vi "PV reconnect.vi"(10 "Input cluster":T1) -> (0 "Vlim":bool, 1 "flim":bool, 2 "failure_flag 3":bool)   [LabVIEW 2016]
uses:
  Communication/Global communication.vi
  Communication/Global communication output.vi
panel:
  out "ready? 2":bool
  out "Boolean":bool
  in  "Max_2":bool
  in  "Max_2":bool
  in  "Max_1":bool
  in  "Max?":bool
  in  "Vlim?":bool
  in  "flim?":bool
  in  "ready?":bool
  in  "i>=20?":bool
  in  "=1?":bool
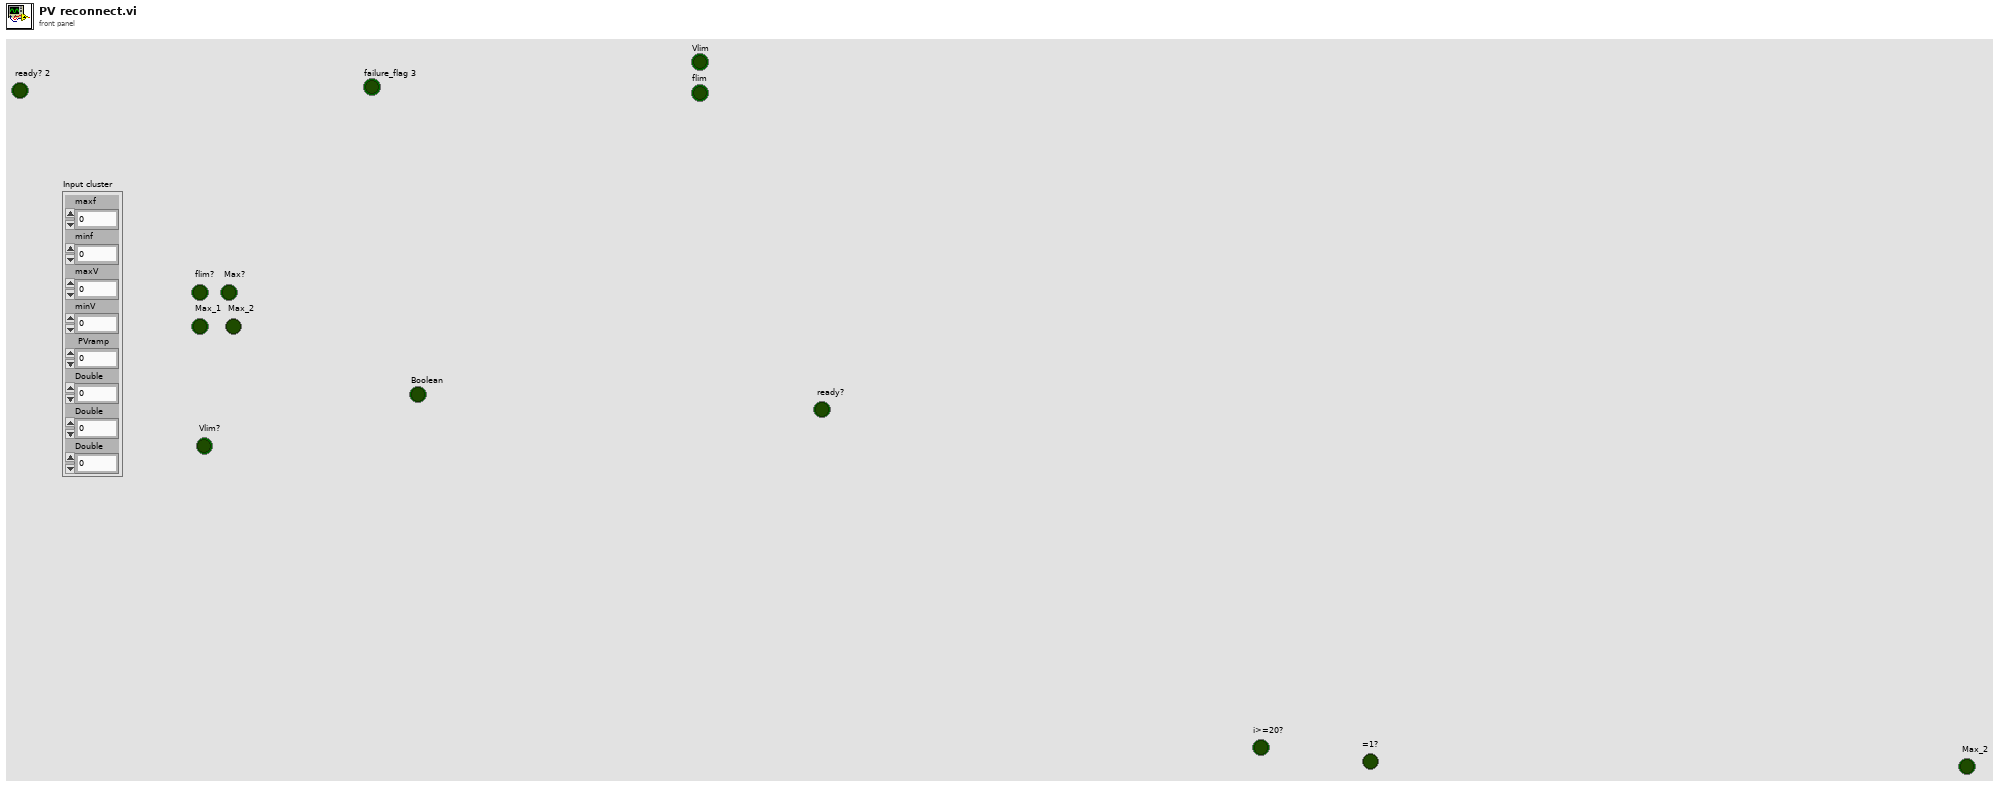
[diagram p1: front panel]
types:
  T1 = cluster{"maxf":dbl, "minf":dbl, "maxV":dbl, "minV":dbl, " PVramp":dbl, "Double":dbl, "Double":dbl, "Double":dbl}
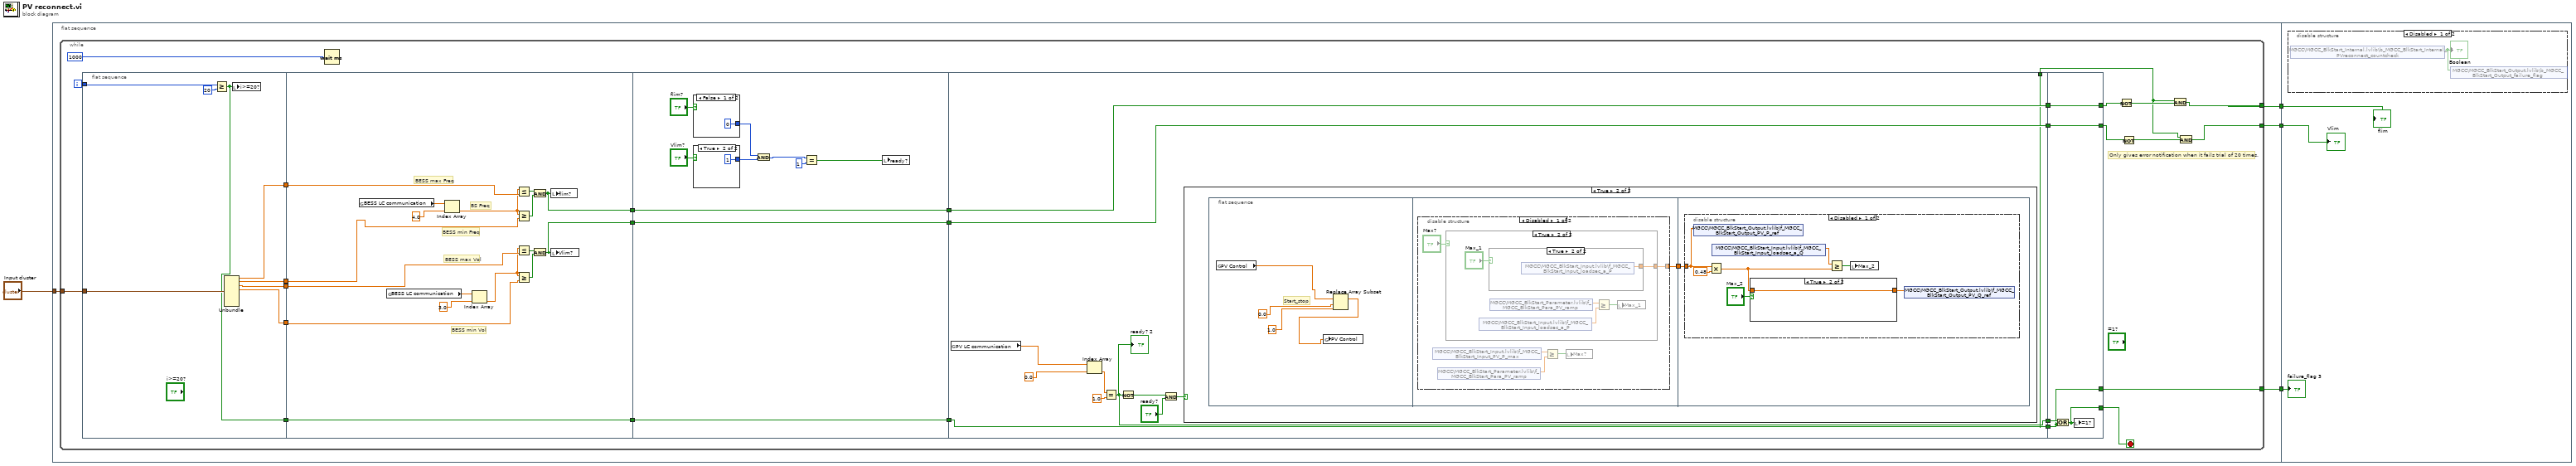
[diagram p0: block diagram]
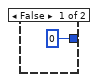
[diagram p2: hidden frame]
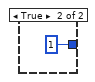
[diagram p3: hidden frame]
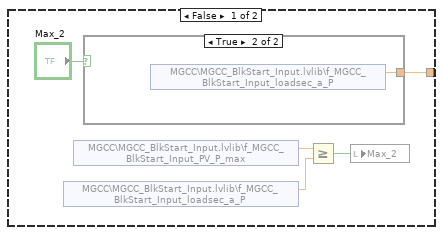
[diagram p5: hidden frame]
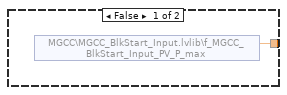
[diagram p6: hidden frame]
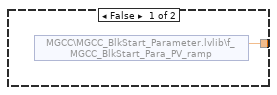
[diagram p7: hidden frame]
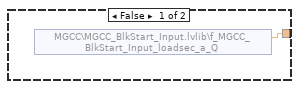
[diagram p9: hidden frame]
diagram:
  n1 = flat-sequence {
    tunnel: [w8] -> w4
    tunnel: "Input cluster" -> [w7]
    tunnel: [w6] -> w2
    tunnel: [w5] -> w1
    tunnel: w4 -> [w128]
    tunnel: w2 -> [w126]
    tunnel: w1 -> [w127]
    frame #0 {
      n2 = while {
        tunnel: [w31] -> w8
        tunnel: w7 -> [w30]
        tunnel: [w15] -> w6
        tunnel: [w14] -> w5
        i -> [w34]
        stop <- w17 stop-if-true
        # "Only gives error notification when it fails trial of 20 times."
        n3 = flat-sequence {
          tunnel: w34 -> [w43]
          tunnel: w30 -> [w41]
          tunnel: [w40] -> w29
          tunnel: [w39] -> w28
          tunnel: [w38] -> w27
          tunnel: [w37] -> w26
          tunnel: [w36] -> w16
          tunnel: [w60] -> w23
          tunnel: w29 -> [w55]
          tunnel: w28 -> [w54]
          tunnel: w27 -> [w53]
          tunnel: w26 -> [w52]
          tunnel: [w51] -> w21
          tunnel: [w50] -> w19
          tunnel: w16 -> [w60]
          tunnel: w23 -> [w70]
          tunnel: [w70] -> w22
          tunnel: w21 -> [w69]
          tunnel: [w69] -> w20
          tunnel: w19 -> [w68]
          tunnel: [w68] -> w18
          tunnel: w22 -> [w75]
          tunnel: [w75] -> w33
          tunnel: [w81] -> w32
          tunnel: w20 -> [w80]
          tunnel: w18 -> [w79]
          tunnel: [w80] -> w25
          tunnel: [w79] -> w24
          tunnel: [w75] -> w9
          tunnel: w33 -> [w124]
          tunnel: w32 -> [w125]
          tunnel: [w124] -> w31
          tunnel: [w123] -> w13
          tunnel: w25 -> [w123]
          tunnel: [w122] -> w11
          tunnel: w24 -> [w122]
          tunnel: [w121] -> w17
          frame #0 {
            n4 = Greater Or Equal?(x=w43, y=20) -> (x >= y?=w36:bool)
            n5 = Unbundle(w41) -> ("maxf"=w40:dbl, "minf"=w39:dbl, "maxV"=w38:dbl, "minV"=w37:dbl)  [unwired: 4 out]
            n6 = local write "i>=20?"(w36) -> ()
          }
          frame #1 {
            # "BESS min Vol"
            # "BESS max Vol"
            # "BESS min Freq"
            # "BS Freq"
            # "BESS max Freq"
            n7 = global read "Global communication.vi" "BESS LC communication"() -> (w49:dbl[])
            n8 = global read "Global communication.vi" "BESS LC communication"() -> (w46:dbl[])
            n9 = Index Array(array=w49, index=4.0) -> (element=w47:dbl)
            n10 = Index Array(array=w46, index=3.0) -> (element=w45:dbl)
            n11 = Less Or Equal?(x=w47, y=w55) -> (x <= y?=w59:bool)
            n12 = Greater Or Equal?(x=w47, y=w54) -> (x >= y?=w58:bool)
            n13 = Less Or Equal?(x=w45, y=w53) -> (x <= y?=w57:bool)
            n14 = Greater Or Equal?(x=w45, y=w52) -> (x >= y?=w56:bool)
            n15 = And(x=w59, y=w58) -> (x .and. y?=w51:bool)
            n16 = And(x=w57, y=w56) -> (x .and. y?=w50:bool)
            n17 = local write "flim?"(w51) -> ()
            n18 = local write "Vlim?"(w50) -> ()
          }
          frame #2 {
            n19 = case shown="False" "flim?" {
              tunnel: [0 1] -> w66
              frame False {
              }
              frame True {
              }
            }
            n20 = case shown="True" "Vlim?" {
              tunnel: [0 1] -> w67
              frame False {
              }
              frame True {
              }
            }
            n21 = And(x=w66, y=w67) -> (x .and. y?=w61:i32)
            n22 = Equal?(x=w61, y=1) -> (x = y?=w63:bool)
            n23 = local write "ready?"(w63) -> ()
          }
          frame #3 {
            n24 = global read "Global communication.vi" "PV LC communication"() -> (w76:dbl[])
            n25 = Index Array(array=w76, index=0.0) -> (element=w77:dbl)
            n26 = Equal?(x=w77, y=1.0) -> (x = y?=w81:bool)
            "ready? 2" <- w81
            n27 = Not(x=w81) -> (.not. x?=w83:bool)
            n28 = And(x=w83, y="ready?") -> (x .and. y?=w84:bool)
            n29 = case shown="True" w84 {
              frame False {
              }
              frame True {
                n30 = flat-sequence {
                  tunnel: [w91] -> w86
                  tunnel: w86 -> [w111]
                  frame #0 {
                    # "Start_stop"
                    n31 = global read "Global communication output.vi" "PV Control"() -> (w88:dbl[])
                    n32 = Replace Array Subset(array=w88, new element=1.0, index=0.0) -> (w87:dbl[])
                    n33 = global write "Global communication output.vi" "PV Control"(w87) -> ()
                  }
                  frame #1 {
                    n34 = disable-structure shown="Disabled" {
                      disable-tunnel: [w92 _] -> w91
                      frame Disabled {
                        n35 = shared-variable "MGCC\\MGCC_BlkStart_Input.lvlib\\f_MGCC_BlkStart_Input_PV_P_max"() -> (w96:dbl)  [unwired: 1 in, 1 out]
                        n36 = shared-variable "MGCC\\MGCC_BlkStart_Parameter.lvlib\\f_MGCC_BlkStart_Para_PV_ramp"() -> (w95:dbl)  [unwired: 1 in, 1 out]
                        n37 = case shown="True" "Max?" {
                          tunnel: [w97 w104] -> w92
                          frame False {
                            n38 = shared-variable "MGCC\\MGCC_BlkStart_Input.lvlib\\f_MGCC_BlkStart_Input_loadsec_a_P"() -> (w100:dbl)  [unwired: 1 in, 1 out]
                            n39 = shared-variable "MGCC\\MGCC_BlkStart_Input.lvlib\\f_MGCC_BlkStart_Input_PV_P_max"() -> (w98:dbl)  [unwired: 1 in, 1 out]
                            n40 = case shown="True" "Max_2" {
                              tunnel: [w102 w103] -> w97
                              frame False {
                                n41 = shared-variable "MGCC\\MGCC_BlkStart_Input.lvlib\\f_MGCC_BlkStart_Input_PV_P_max"() -> (w102:dbl)  [unwired: 1 in, 1 out]
                              }
                              frame True {
                                n42 = shared-variable "MGCC\\MGCC_BlkStart_Input.lvlib\\f_MGCC_BlkStart_Input_loadsec_a_P"() -> (w103:dbl)  [unwired: 1 in, 1 out]
                              }
                            }
                            n43 = Greater Or Equal?(x=w98, y=w100) -> (x >= y?=w101:bool)
                            n44 = local write "Max_2"(w101) -> ()
                          }
                          frame True {
                            n45 = shared-variable "MGCC\\MGCC_BlkStart_Input.lvlib\\f_MGCC_BlkStart_Input_loadsec_a_P"() -> (w106:dbl)  [unwired: 1 in, 1 out]
                            n46 = case shown="True" "Max_1" {
                              tunnel: [w109 w110] -> w104
                              frame False {
                                n47 = shared-variable "MGCC\\MGCC_BlkStart_Parameter.lvlib\\f_MGCC_BlkStart_Para_PV_ramp"() -> (w109:dbl)  [unwired: 1 in, 1 out]
                              }
                              frame True {
                                n48 = shared-variable "MGCC\\MGCC_BlkStart_Input.lvlib\\f_MGCC_BlkStart_Input_loadsec_a_P"() -> (w110:dbl)  [unwired: 1 in, 1 out]
                              }
                            }
                            n49 = shared-variable "MGCC\\MGCC_BlkStart_Parameter.lvlib\\f_MGCC_BlkStart_Para_PV_ramp"() -> (w107:dbl)  [unwired: 1 in, 1 out]
                            n50 = Greater Or Equal?(x=w107, y=w106) -> (x >= y?=w108:bool)
                            n51 = local write "Max_1"(w108) -> ()
                          }
                        }
                        n52 = Greater Or Equal?(x=w96, y=w95) -> (x >= y?=w94:bool)
                        n53 = local write "Max?"(w94) -> ()
                      }
                      frame Enabled {
                      }
                    }
                  }
                  frame #2 {
                    n54 = disable-structure shown="Disabled" {
                      disable-tunnel: w111 -> [w117 _]
                      frame Disabled {
                        n55 = shared-variable "MGCC\\MGCC_BlkStart_Output.lvlib\\f_MGCC_BlkStart_Output_PV_P_ref"(w117) -> ()  [unwired: 1 in, 1 out]
                        n56 = Multiply(x=w117, y=0.48) -> (x*y=w113:dbl)
                        n57 = shared-variable "MGCC\\MGCC_BlkStart_Input.lvlib\\f_MGCC_BlkStart_Input_loadsec_a_Q"() -> (w116:dbl)  [unwired: 1 in, 1 out]
                        n58 = case shown="True" "Max_2" {
                          tunnel: w113 -> [_ w120]
                          tunnel: [w119 w120] -> w112
                          frame False {
                            n59 = shared-variable "MGCC\\MGCC_BlkStart_Input.lvlib\\f_MGCC_BlkStart_Input_loadsec_a_Q"() -> (w119:dbl)  [unwired: 1 in, 1 out]
                          }
                          frame True {
                          }
                        }
                        n60 = Greater Or Equal?(x=w116, y=w113) -> (x >= y?=w115:bool)
                        n61 = local write "Max_2"(w115) -> ()
                        n62 = shared-variable "MGCC\\MGCC_BlkStart_Output.lvlib\\f_MGCC_BlkStart_Output_PV_Q_ref"(w112) -> ()  [unwired: 1 in, 1 out]
                      }
                      frame Enabled {
                      }
                    }
                  }
                }
              }
            }
          }
          frame #4 {
            n63 = Or(x=w125, y=w124) -> (x .or. y?=w121:bool)
            n64 = local write "=1?"(w121) -> ()
          }
        }
        n65 = Wait (ms)(milliseconds to wait=1000) -> ()  [unwired: 1 out]
        n66 = Not(x=w13) -> (.not. x?=w12:bool)
        n67 = Not(x=w11) -> (.not. x?=w10:bool)
        n68 = And(x=w9, y=w12) -> (x .and. y?=w15:bool)
        n69 = And(x=w9, y=w10) -> (x .and. y?=w14:bool)
      }
    }
    frame #1 {
      n70 = disable-structure shown="Disabled" {
        frame Disabled {
          n71 = shared-variable "MGCC\\MGCC_BlkStart_Internal.lvlib\\b_MGCC_BlkStart_Internal_PVreconnect_countcheck"() -> (w129:bool)  [unwired: 1 in, 1 out]
          "Boolean" <- w129
          n72 = shared-variable "MGCC\\MGCC_BlkStart_Output.lvlib\\b_MGCC_BlkStart_Output_failure_flag"(w129) -> ()  [unwired: 1 in, 1 out]
        }
        frame Enabled {
        }
      }
      "failure_flag 3" <- w128
      "Vlim" <- w127
      "flim" <- w126
    }
  }
